vi "HilitePicture__LCR.vi"(8 "error in (no error)":errorcluster, 9 "Percentage(30)":dbl=30.0, 11 "image data":T1) -> (0 "error out":errorcluster, 3 "Hilited Picture":T1)   [LabVIEW 2011, in "BooleanXControl__LCR.xctl"]
doc: "This VI hilites a picture"
uses:
  BooleanXControl__LCR.xctl
  <vilib>/picture/picture.llb/imagedata.ctl
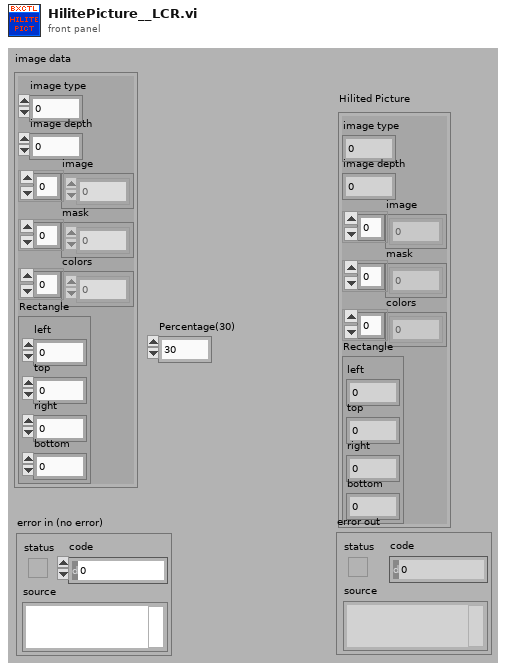
[diagram p1: front panel]
types:
  T1 = typedef "imagedata.ctl" = cluster{"image type":i32, "image depth":i32, "image":u8[], "mask":u8[], "colors":u32[], "Rectangle":cluster{"left":i16, "top":i16, "right":i16, "bottom":i16}}
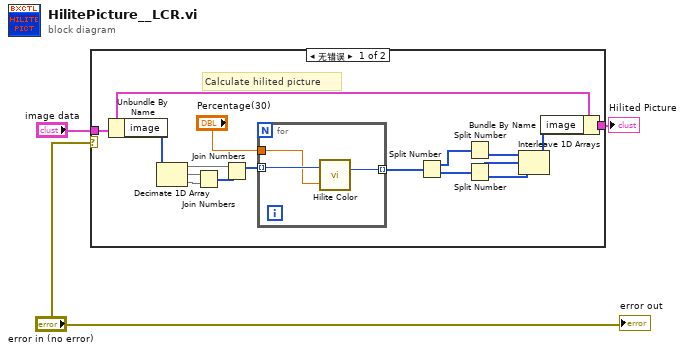
[diagram p0: block diagram]
diagram:
  n1 = case shown="无错误" "error in (no error)" {
    tunnel: "image data" -> [w6 w23]
    tunnel: [w5 w23] -> w2
    frame No Error {
      # "Calculate hilited picture"
      n2 = Unbundle By Name(w6) -> ("image"=w8:u8[])
      n3 = Decimate 1D Array(w8) -> (w16:u8[], w19:u8[], w18:u8[])
      n4 = Join Numbers(hi=w19, lo=w18) -> ((hi.lo)=w17:u16[])
      n5 = Join Numbers(hi=w16, lo=w17) -> ((hi.lo)=w7:u32[])
      n6 = for {
        tunnel: w7 -> [w21] mode=indexing
        tunnel: [w22] -> w15 mode=indexing
        tunnel: "Percentage(30)" -> [w20]
        n7 = call <vilib>:"Hilite Color.vi"("Percentage(30)"=w20, "Color In"=w21) -> ("Hilite"=w22:u32)  [unwired: 1 out]
      }
      n8 = Split Number(x=w15) -> (hi(x)=w14:u16[], lo(x)=w13:u16[])
      n9 = Split Number(x=w14) -> (lo(x)=w12:u8[])  [unwired: 1 out]
      n10 = Split Number(x=w13) -> (hi(x)=w11:u8[], lo(x)=w10:u8[])
      n11 = Interleave 1D Arrays(w12, w11, w10) -> (w9:u8[])
      n12 = Bundle By Name(cluster=w6, "image"=w9) -> (w5:T1)
    }
    frame Error {
    }
  }
  "Hilited Picture" <- w2
  "error out" <- "error in (no error)"
